vi "Disable Measurements.vi"(0 "Register Buses":refnum<class "ni579x Register Bus v1 Host.lvclass">[](array[class]), 11 "error in":errorcluster) -> (4 "Register Buses (out)":refnum<class "ni579x Register Bus v1 Host.lvclass">[](array[class]), 15 "error out":errorcluster)   [LabVIEW 2012, in "ni579x Synchronization v1 Host.lvlib"]
doc: "Turn off the measurement circuits on the FPGA."
uses:
  <instrlib>/ni579x/Synchronization/v1/Host/ni579x Synchronization v1 Host.lvlib
  <instrlib>/ni579x/Register Bus/v1/Host/ni579x Register Bus v1 Host.lvclass
  <instrlib>/ni579x/Synchronization/v1/Shared/ni579x Synchronization Register Addresses.ctl
  <instrlib>/ni579x/Register Bus/v1/Host/Public/Register Write.ctl
  <instrlib>/ni579x/Config/v1/Shared/Types/ni579x Register Bus Subsystem ID.ctl
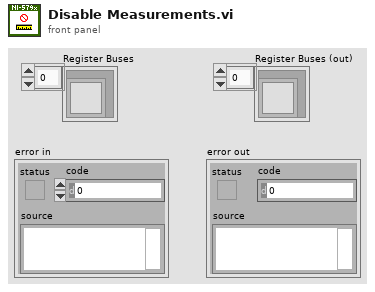
[diagram p1: front panel]
types:
  T1 = typedef "ni579x Register Bus Subsystem ID.ctl" = u8
  T2 = typedef "ni579x Register Bus v1 Host.lvclass/Register Write.ctl" = cluster{"subsystem":u8, "address":u16, "data":u32}
  T3 = typedef "ni579x Synchronization Register Addresses.ctl" = enum16{"Signature", "Current Version", "Oldest Compatible Version", "Scratch Register", "sync.master", "sync.meas.enable", "sync.meas.ready", "sync.meas.arm", "sync.meas.valid", "sync.meas.value", "sync.cptr.adjust", "sync.cptr.period", "sync.meas.oversample factor"}
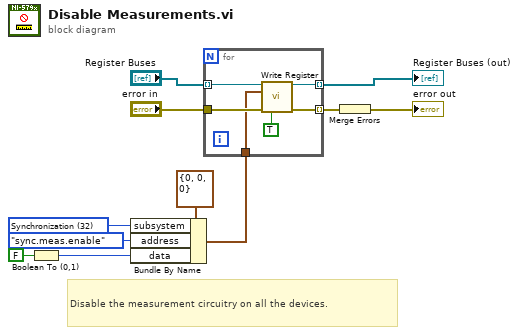
[diagram p0: block diagram]
diagram:
  w9 = T1 32 items=["FAM Register Operation"=0, "User Command"=16, "Synchronization"=32] ("Subsystem ID")
  # "Disable the measurement circuitry on all the devices."
  n1 = Boolean To (0,1)(Boolean=FALSE ("sync.Master")) -> (0, 1=w11:i16)
  n2 = Bundle By Name(cluster=T2 {"subsystem"=0, "address"=0, "data"=0} ("register write"), "subsystem"=w9, "address"=ni579x_Synchronization_Register_Addresses."sync.meas.enable" ("Synchronization Registers"), "data"=w11) -> (w6:T2)
  n3 = for {
    tunnel: "Register Buses" -> [w17] mode=indexing
    tunnel: w6 -> [w15]
    tunnel: [w13] -> w1 mode=indexing
    tunnel: "error in" -> [w16]
    tunnel: [w12] -> w3 mode=indexing
    n4 = call <instrlib>:"Write Register.vi"("session in"=w17, "register write"=w15, "error in"=w16, "wait until committed"=TRUE) -> ("session out"=w13:refnum<class "ni579x Register Bus v1 Host.lvclass">, "error out"=w12:errorcluster)  [unwired: 10 in]
  }
  "Register Buses (out)" <- w1
  n5 = Merge Errors(w3) -> (→"error out":errorcluster)
